vi "CommonVIs_EnumsToStrings.vi"(1 "ArrayEnumVariantIn":variant, 2 "SingleEnumVariantIn":variant, 5 "error in (no error)":errorcluster) -> (15 "EnumItems(string)":string[](array[string]), 16 "EnumItem":string, 17 "EnumChoices":string[](array[string]), 19 "error out":errorcluster)   [LabVIEW 2014]
doc: "Uses a flatten XML string of a Enum-type <B>\"XmlEnumStringIn\"</B> to find the acctually value of the enum.\nThis is normally used when a Enum has been flatten to a variant.\nIt could also take the enum variant as an input\nIt the Variant ENUM is of string type it will send it through without any errors"
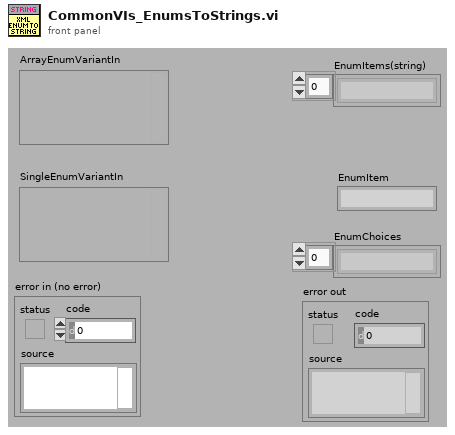
[diagram p1: front panel]
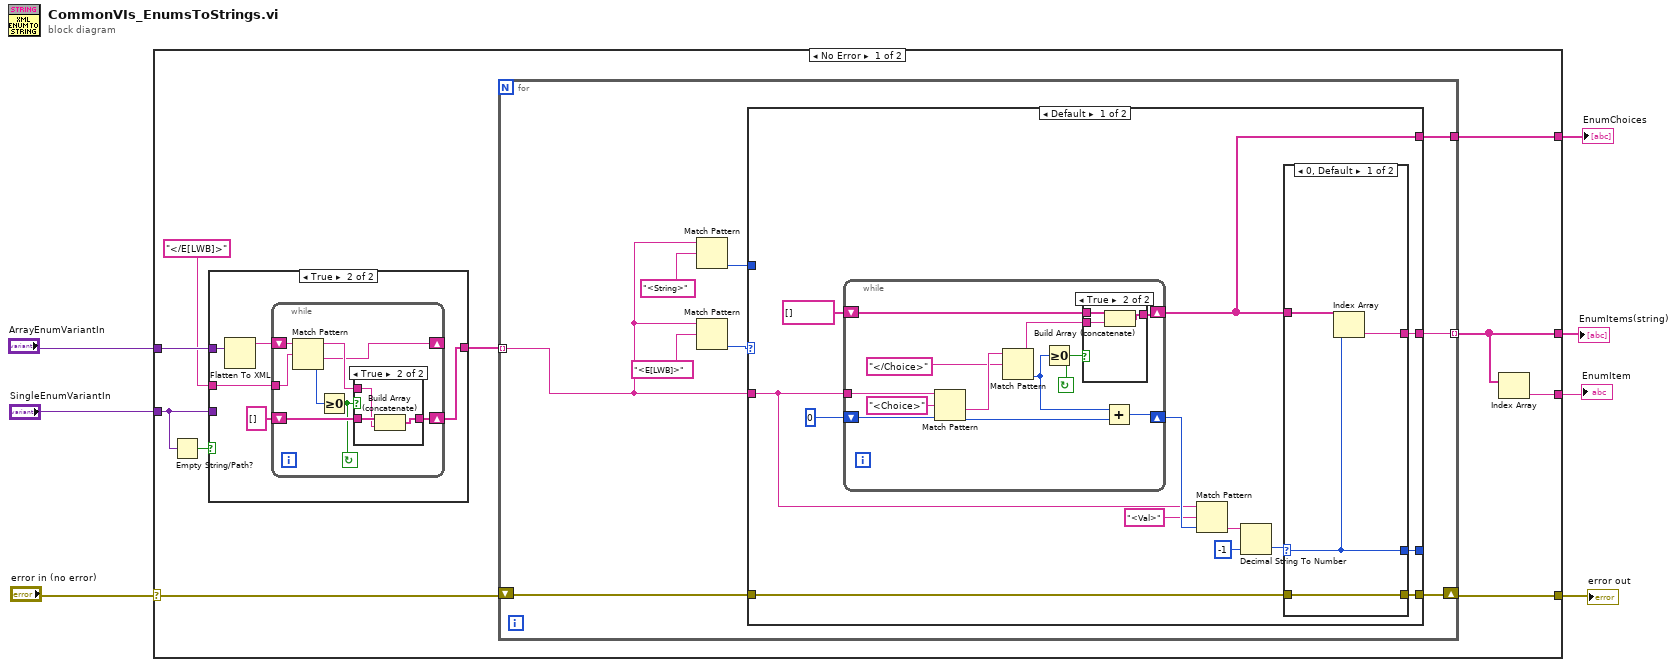
[diagram p0: block diagram]
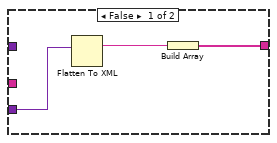
[diagram p2: hidden frame]
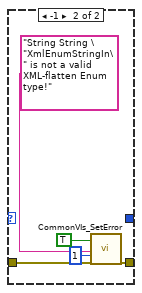
[diagram p4: hidden frame]
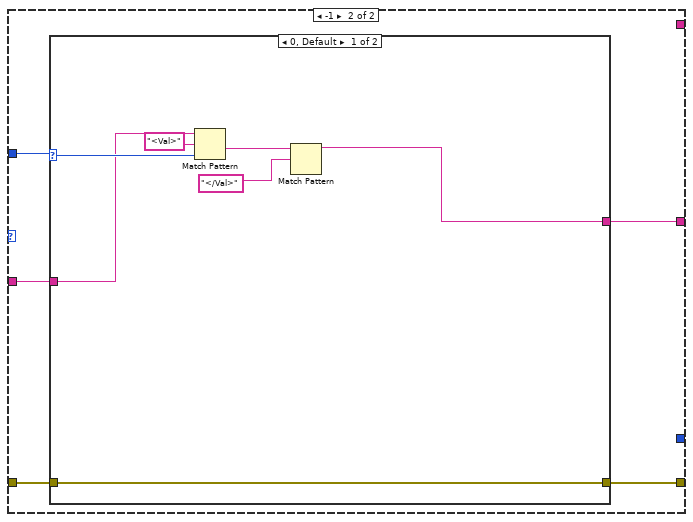
[diagram p6: hidden frame]
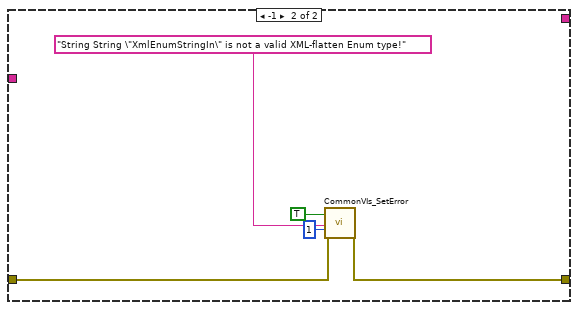
[diagram p7: hidden frame]
diagram:
  n1 = case shown="No Error" "error in (no error)" {
    selector: "error in (no error)" -> [w14 w102]
    tunnel: [w17 w102] -> w4
    tunnel: [w16 _] -> w5
    tunnel: "ArrayEnumVariantIn" -> [w10 _]
    tunnel: [w15 _] -> w3
    tunnel: "SingleEnumVariantIn" -> [w11 _]
    tunnel: [w8 _] -> w1
    frame No Error {
      n2 = Empty String/Path?(string/path=w11) -> (empty?=w13:bool)
      n3 = case shown="True" w13 {
        tunnel: w11 -> [w20 _]
        tunnel: [w18 w21] -> w12
        tunnel: w10 -> [_ w25]
        tunnel: "</E[LWB]>" ("regular expression") -> [_ w23]
        frame False {
          n4 = Flatten To XML(anything=w20) -> (xml string=w19:string)
          n5 = Build Array(w19) -> (w18:string[])
        }
        frame True {
          n6 = Flatten To XML(anything=w25) -> (xml string=w24:string)
          n7 = while {
            shift-right: [w26] -> _
            shift-left: w24 -> [w33]
            tunnel: w23 -> [w32]
            shift-right: [w29] -> w21
            shift-left: string[] [] -> [w30]
            stop <- w28 continue-if-true
            n8 = Match Pattern(string=w33, regular expression=w32) -> (before substring=w27:string, after substring=w26:string, offset past match=w31:i32)  [unwired: 2 out]
            n9 = Greater Or Equal To 0?(x=w31) -> (x >= 0?=w28:bool)
            n10 = case shown="True" w28 {
              tunnel: w30 -> [w34 w37]
              tunnel: [w34 w36] -> w29
              tunnel: w27 -> [_ w35]
              frame False {
              }
              frame True {
                n11 = Build Array (concatenate)(w37, w35) -> (w36:string[])
              }
            }
          }
        }
      }
      n12 = for {
        tunnel: [w44] -> w16 mode=indexing
        tunnel: w12 -> [w39] mode=indexing
        shift-right: [w41] -> w17
        shift-left: w14 -> [w40]
        tunnel: [w38] -> w8
        n13 = Match Pattern(string=w39, regular expression="<String>") -> (offset past match=w42:i32)  [unwired: 4 out]
        n14 = Match Pattern(string=w39, regular expression="<E[LWB]>") -> (offset past match=w45:i32)  [unwired: 4 out]
        n15 = case shown="Default" w45 {
          tunnel: w39 -> [w56 w85]
          tunnel: w40 -> [w51 w89]
          tunnel: [w50 w88] -> w41
          tunnel: [w49 w86] -> w44
          tunnel: [w48 _] -> _
          tunnel: w42 -> [_ w87]
          tunnel: [w47 _] -> w38
          frame Default {
            n16 = while {
              shift-left: 0 ("offset past match") -> [w78]
              shift-right: [w74] -> w57
              tunnel: w56 -> [w79]
              shift-right: [w70] -> w47
              shift-left: string[] [] -> [w71]
              stop <- w72 continue-if-true
              n17 = Match Pattern(string=w79, regular expression="<Choice>", offset (0)=w78) -> (after substring=w77:string, offset past match=w75:i32)  [unwired: 2 out]
              n18 = Match Pattern(string=w77, regular expression="</Choice>") -> (before substring=w69:string, offset past match=w73:i32)  [unwired: 3 out]
              n19 = Greater Or Equal To 0?(x=w73) -> (x >= 0?=w72:bool)
              n20 = case shown="True" w72 {
                tunnel: w71 -> [w81 w84]
                tunnel: [w81 w83] -> w70
                tunnel: w69 -> [_ w82]
                frame False {
                }
                frame True {
                  n21 = Build Array (concatenate)(w84, w82) -> (w83:string[])
                }
              }
              n22 = Add(x=w73, y=w75) -> (x+y=w74:i32)
            }
            n23 = Match Pattern(string=w56, regular expression="<Val>", offset (0)=w57) -> (after substring=w54:string)  [unwired: 3 out]
            n24 = Decimal String To Number(string=w54, default (0L)=-1 ("default (0 I32)")) -> (number=w52:i32)  [unwired: 2 out]
            n25 = case shown="0, Default" w52 {
              selector: w52 -> [w60 _]
              tunnel: w51 -> [w63 w65]
              tunnel: [w63 w64] -> w50
              tunnel: w47 -> [w62 _]
              tunnel: [w61 _] -> w49
              tunnel: [w60 _] -> w48
              frame 0, Default {
                n26 = Index Array(array=w62, index=w60) -> (element=w61:string)
              }
              frame -1 {
                n27 = call <resource>:"CommonVIs_SetError.vi"("status"=TRUE, "code (5000)"=1, "source"="String String \"XmlEnumStringIn\" is not a valid XML-flatten Enum type!", "error in (no error)"=w65) -> ("error out"=w64:errorcluster)  [unwired: 1 in, 14 out]
              }
            }
          }
          frame -1 {
            n28 = case shown="0, Default" w87 {
              selector: w87 -> [w95 _]
              tunnel: w89 -> [w91 w101]
              tunnel: [w91 w100] -> w88
              tunnel: [w92 _] -> w86
              tunnel: w85 -> [w90 _]
              frame 0, Default {
                n29 = Match Pattern(string=w90, regular expression="<Val>", offset (0)=w95) -> (after substring=w94:string)  [unwired: 3 out]
                n30 = Match Pattern(string=w94, regular expression="</Val>") -> (before substring=w92:string)  [unwired: 4 out]
              }
              frame -1 {
                n31 = call <resource>:"CommonVIs_SetError.vi"("status"=TRUE, "code (5000)"=1, "source"="String String \"XmlEnumStringIn\" is not a valid XML-flatten Enum type!", "error in (no error)"=w101) -> ("error out"=w100:errorcluster)  [unwired: 1 in, 14 out]
              }
            }
          }
        }
      }
      n32 = Index Array(array=w16) -> (element=w15:string)  [unwired: 1 in]
    }
    frame Error {
    }
  }
  "error out" <- w4
  "EnumItems(string)" <- w5
  "EnumItem" <- w3
  "EnumChoices" <- w1
